vi "Read SV_Publisher.vi"(11 "Device in":refnum<class "Device.lvclass">) -> (2 "SV_Publisher.lvclass":refnum<class "SV_Publisher.lvclass">)   [LabVIEW 2019, in "Device.lvclass"]
uses:
  Device.lvclass
  SV_Puplisher_class/SV_Publisher.lvclass
  Device.lvclass/Device.ctl
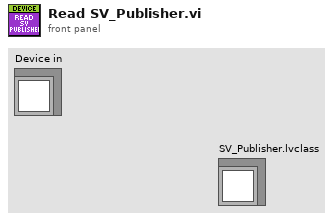
[diagram p1: front panel]
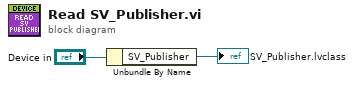
[diagram p0: block diagram]
diagram:
  n1 = Unbundle By Name("Device in") -> ("SV_Publisher"=→"SV_Publisher.lvclass":refnum<class "SV_Publisher.lvclass">)
